vi "KonstruiereScanSteuerung.vi"(0 "VektorCluster":T2={"StartPunkt [m]"={"x"=-0.0005000005000000012, "y"=-0.0005000005000000081}, "ZeilenIncrement [m]"={"x"=0.0, "y"=0.0001}, "Zeile [m/s]"={"x"=1.0, "y"=0.0}, "Zeit/Zeile [s]"=0.001}, 1 "ParameterCluster":T4={"x Pixel"=250, "Lines"=250, "Bidirektional"=TRUE, "AD-Frequency [Hz]"=4000000.0, "Galvo Cycle [s]"=1e-05, "Smartmovedelay [s]"=0.00119, "max.accel. [m/s^2]"=270000.0}) -> (2 "ScanSteuerung":T3(array[cluster])=[{"Zeitpunkt [s]"=0.0, "Wirkung"=enum."Abs", "Kanal"=enum."SMoveTime", "Wert (/s)"=0.0008}, {"Zeitpunkt [s]"=0.0, "Wirkung"=enum."Abs", "Kanal"=enum."GalvoX", "Wert (/s)"=-0.0005000005000000012}, {"Zeitpunkt [s]"=0.0, "Wirkung"=enum."Abs", "Kanal"=enum."GalvoY", "Wert (/s)"=-0.0005000005000000081}, {"Zeitpunkt [s]"=0.0, "Wirkung"=enum."Abs", "Kanal"=enum."Galvo3", "Wert (/s)"=0.0}, {"Zeitpunkt [s]"=0.0, "Wirkung"=enum."LoopStart", "Kanal"=enum."Loop", "Wert (/s)"=10.0}, {"Zeitpunkt [s]"=0.0, "Wirkung"=enum."Inc", "Kanal"=enum."GalvoX", "Wert (/s)"=0.10000010000000015}, {"Zeitpunkt [s]"=0.0, "Wirkung"=enum."Inc", "Kanal"=enum."GalvoY", "Wert (/s)"=0.0}, {"Zeitpunkt [s]"=0.0, "Wirkung"=enum."Inc", "Kanal"=enum."Galvo3", "Wert (/s)"=51200.0}, {"Zeitpunkt [s]"=0.01, "Wirkung"=enum."Abs", "Kanal"=enum."Digital", "Wert (/s)"=1.0}, {"Zeitpunkt [s]"=0.01, "Wirkung"=enum."Inc", "Kanal"=enum."GalvoX", "Wert (/s)"=0.0}, {"Zeitpunkt [s]"=0.01, "Wirkung"=enum."Inc", "Kanal"=enum."GalvoY", "Wert (/s)"=0.6250006249999993}, {"Zeitpunkt [s]"=0.01, "Wirkung"=enum."Inc", "Kanal"=enum."Galvo3", "Wert (/s)"=0.0}, {"Zeitpunkt [s]"=0.01008, "Wirkung"=enum."Abs", "Kanal"=enum."Digital", "Wert (/s)"=0.0}, {"Zeitpunkt [s]"=0.01008, "Wirkung"=enum."Inc", "Kanal"=enum."GalvoX", "Wert (/s)"=-0.10000010000000015}, {"Zeitpunkt [s]"=0.01008, "Wirkung"=enum."Inc", "Kanal"=enum."GalvoY", "Wert (/s)"=-0.0}, {"Zeitpunkt [s]"=0.01008, "Wirkung"=enum."Inc", "Kanal"=enum."Galvo3", "Wert (/s)"=-51200.0}, {"Zeitpunkt [s]"=0.02008, "Wirkung"=enum."Abs", "Kanal"=enum."Digital", "Wert (/s)"=1.0}, {"Zeitpunkt [s]"=0.02008, "Wirkung"=enum."Inc", "Kanal"=enum."GalvoX", "Wert (/s)"=0.0}, {"Zeitpunkt [s]"=0.02008, "Wirkung"=enum."Inc", "Kanal"=enum."GalvoY", "Wert (/s)"=0.6250006249999993}, {"Zeitpunkt [s]"=0.02008, "Wirkung"=enum."Inc", "Kanal"=enum."Galvo3", "Wert (/s)"=0.0}, {"Zeitpunkt [s]"=0.02016, "Wirkung"=enum."Abs", "Kanal"=enum."Digital", "Wert (/s)"=0.0}, {"Zeitpunkt [s]"=0.02016, "Wirkung"=enum."LoopEnd", "Kanal"=enum."Loop", "Wert (/s)"=0.0}, {"Zeitpunkt [s]"=0.2016, "Wirkung"=enum."Inc", "Kanal"=enum."GalvoX", "Wert (/s)"=0.0}, {"Zeitpunkt [s]"=0.2016, "Wirkung"=enum."Inc", "Kanal"=enum."GalvoY", "Wert (/s)"=0.0}, {"Zeitpunkt [s]"=0.2016, "Wirkung"=enum."Inc", "Kanal"=enum."Galvo3", "Wert (/s)"=0.0}], 3 "Total time":dbl=0.2016, 4 "Line+Turn [s]":dbl=8e-05 format="%^#_6g")   [LabVIEW 2011]
panel:
  out "Galvo too far":cluster{"x":dbl, "y":dbl}
  out "Galvo too late time":dbl
  out "min Line+turn":dbl
  out "exactTurn [s]":dbl format="%_6g"
  out "AD/pixel":u32
  out "Pixelzeit":dbl
  out "TotalPixel":u16
  out "berechnete Umkehrzeit [s]":dbl=2.8081673263774566e-05 format="%#_4p"
  out "validTotalCycles":u32
  out "ini":T1={"Bitsize-Zwischenbild"=5.5926e-07, "CCDmin"=7850.0, "CCDscale"=-10.85, "GalvoCycle"=1.2e-05, "Ext.AD-clock"=4000000.0, "Steps per optical density"=53.33} {"CCDscale" format="%.2f"; "CCDmin" format="%.2f"; "Bitsize-Zwischenbild" format="%.2e"}
  out "Zeit [s]/zeile":dbl=0.01 min=0.0005 step=0.001 format="%^#_6g"
  out "min SMcycles":u16
  # "Used Units: Pixels or meters in the intermediate image\nchanged May 18 2011\nOld version with straight turn\nPixel,Cycles müssen an jedem Linestart synchron sein\nBerechnet die Umkehrzeit So lange, daß Pixel und SM-Cycle in der nächsten Zeile wieder synchron sind\nbi und unidirektional sind getestet"
  # "fehler: unidirektional lieferz zahlen die Smartmove runden muss: kein12ms raster! fixed??"
  # "TriggerPin0: During Turn: High (Line End)\nTriggerPin1: During Frame: High (Frame Start)"
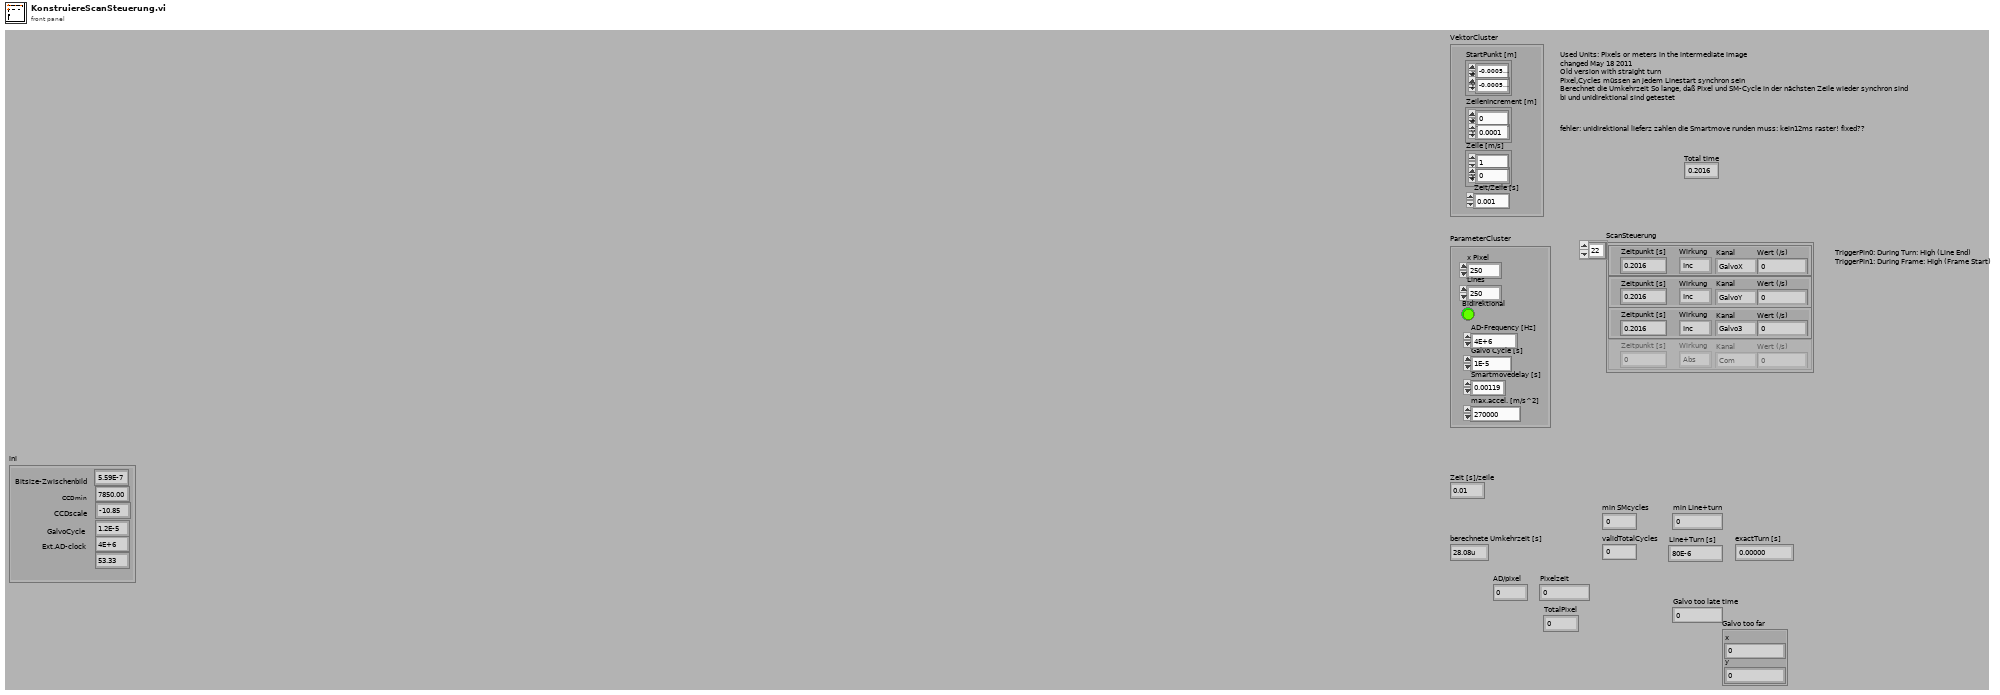
[diagram p1: front panel]
types:
  T1 = cluster{"Bitsize-Zwischenbild":dbl, "CCDmin":dbl, "CCDscale":dbl, "GalvoCycle":dbl, "Ext.AD-clock":dbl, "Steps per optical density":dbl}
  T2 = cluster{"StartPunkt [m]":cluster{"x":dbl, "y":dbl}, "ZeilenIncrement [m]":cluster{"x":dbl, "y":dbl}, "Zeile [m/s]":cluster{"x":dbl, "y":dbl}, "Zeit/Zeile [s]":dbl}
  T3 = cluster{"Zeitpunkt [s]":dbl, "Wirkung":enum16{"Abs", "Rel", "Inc", "IncInc", "LoopStart", "LoopEnd"}, "Kanal":enum16{"Com", "AnalogConfig", "AnalogValue", "GalvoX", "GalvoY", "Galvo3", "Galvo4", "Digital", "Free", "Loop", "SMoveTime", "Image1X", "Image1Y", "Image2X", "Image2Y"}, "Wert (/s)":dbl}[]
  T4 = cluster{"x Pixel":i32, "Lines":i32, "Bidirektional":bool, "AD-Frequency [Hz]":dbl, "Galvo Cycle [s]":dbl, "Smartmovedelay [s]":dbl, "max.accel. [m/s^2]":dbl}
  T5 = enum16{"Com", "AnalogConfig", "AnalogValue", "GalvoX", "GalvoY", "Galvo3", "Galvo4", "Digital", "Free", "Loop", "SMoveTime", "Image1X", "Image1Y", "Image2X", "Image2Y"}
  T6 = enum16{"Abs", "Rel", "Inc", "IncInc", "LoopStart", "LoopEnd"}
  T7 = typedef "ScanControl.ctl" = cluster{"Time [s]":dbl, "action":T8, "channel":T9, "value (/s)":dbl}[]
  T8 = typedef "ScanControl_Action.ctl" = enum16{"Abs", "Rel", "Inc", "IncInc", "LoopStart", "LoopEnd", "WaitTriggerRising"}
  T9 = typedef "ScanControl_Channel.ctl" = enum16{"Com", "AnalogConfig", "AnalogValue", "GalvoX", "GalvoY", "Galvo3", "Galvo4", "Digital", "Free", "Loop", "SMoveTime", "Image1X", "Image1Y", "Image2X", "Image2Y"}
  T10 = cluster{"Ende [s] AD+g raster":dbl, "Wirkung":enum16{"Abs", "Rel", "Inc", "IncInc", "LoopStart", "LoopEnd"}, "Kanal":enum16{"Com", "AnalogConfig", "AnalogValue", "GalvoX", "GalvoY", "Galvo3", "Galvo4", "Digital", "Free", "Loop", "SMoveTime", "Image1X", "Image1Y", "Image2X", "Image2Y"}, dbl}
  T11 = cluster{dbl, "Wirkung":enum16{"Abs", "Rel", "Inc", "IncInc", "LoopStart", "LoopEnd"}, "Kanal":enum16{"Com", "AnalogConfig", "AnalogValue", "GalvoX", "GalvoY", "Galvo3", "Galvo4", "Digital", "Free", "Loop", "SMoveTime", "Image1X", "Image1Y", "Image2X", "Image2Y"}, u8}
  T12 = cluster{dbl, "Wirkung":enum16{"Abs", "Rel", "Inc", "IncInc", "LoopStart", "LoopEnd"}, "Kanal":enum16{"Com", "AnalogConfig", "AnalogValue", "GalvoX", "GalvoY", "Galvo3", "Galvo4", "Digital", "Free", "Loop", "SMoveTime", "Image1X", "Image1Y", "Image2X", "Image2Y"}, dbl}
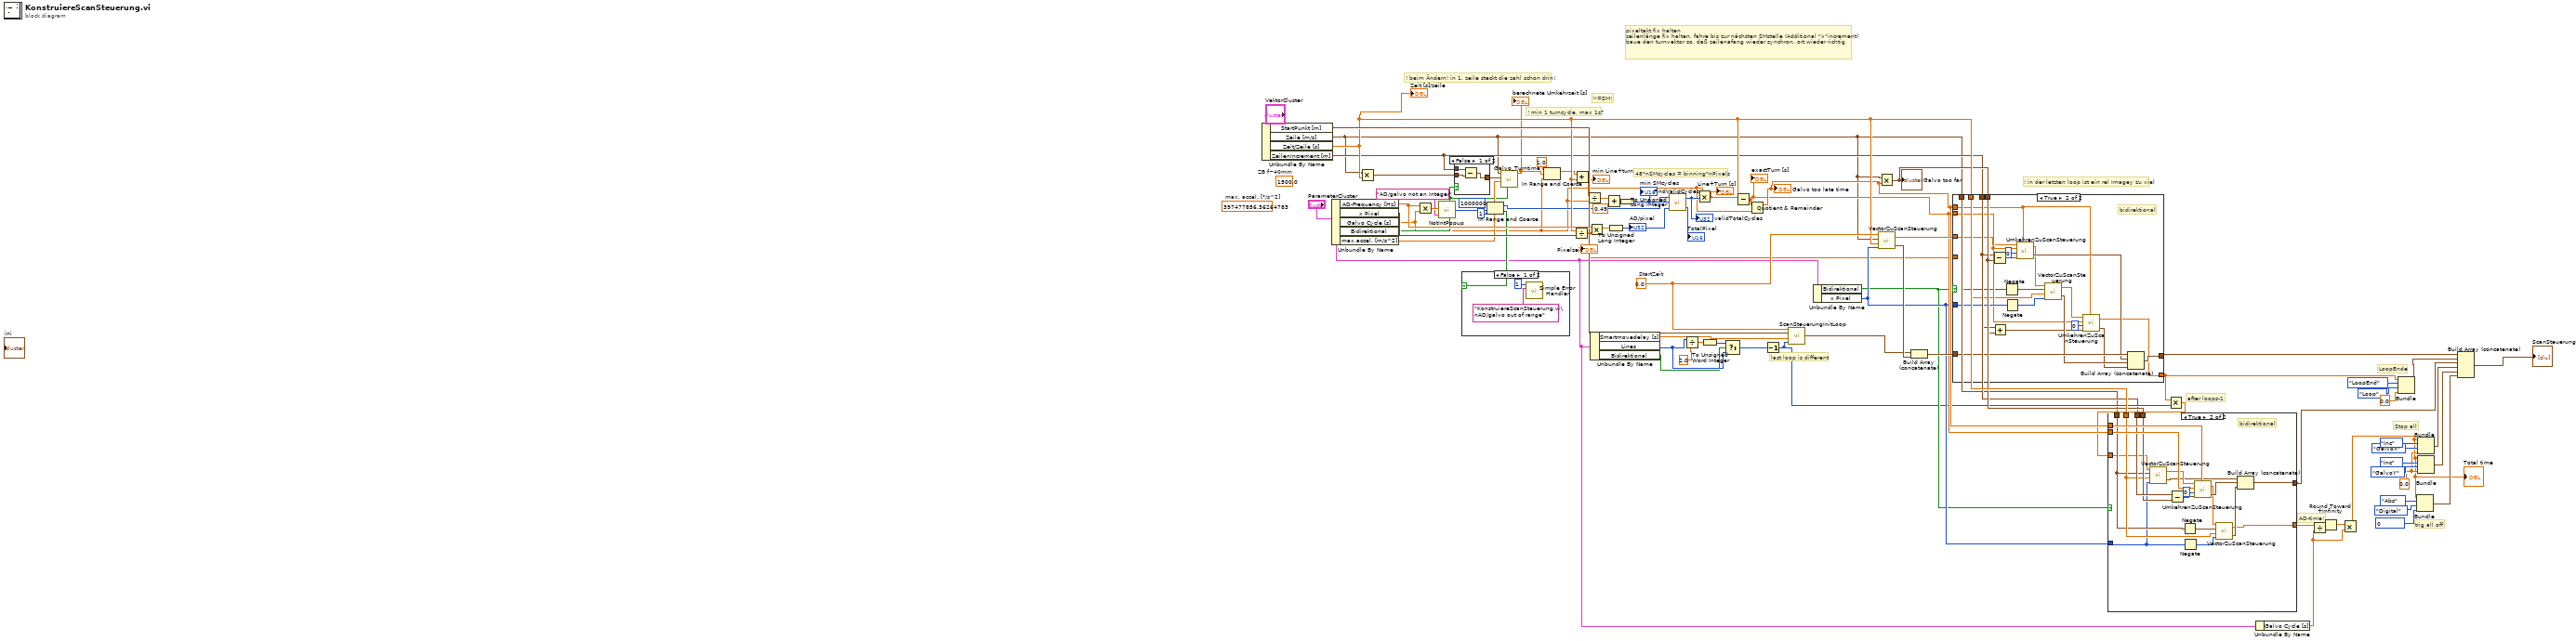
[diagram p0: block diagram]
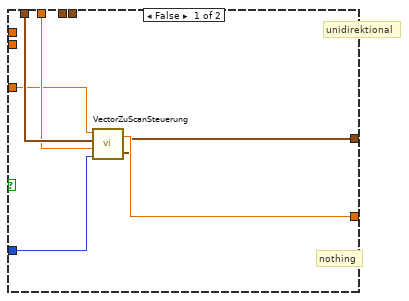
[diagram p3: hidden frame]
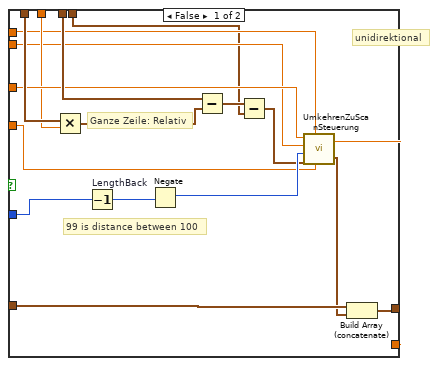
[diagram p5: hidden frame]
diagram:
  (unwired) 397477856.36264783  # max. accel. [°/s^2]
  (unwired) 1500.0  # ZB f~40mm
  w22 = 0.0
  w51 = 0.0  # StartZeit
  # "AD-time!"
  # "after loops-1"
  # "last loop is different"
  # "! in der letzten loop ist ein rel Imagey zu viel"
  # ">=SM!"
  # "! min 1 turncycle, max 1s?"
  # "pixeltakt fix halten\nzeilenlänge fix halten, fahre bis zur nächsten SMstelle (Additional \"x\"increment)\nbaue den turnvektor so, daß zeilenafang wieder synchron, ort wieder richtig"
  # "! beim Ändern! in 1. zeile steckt die zahl schon drin!"
  # "48*nSMcycles = binning*nPixels"
  # "trig all off"
  # "Stop all"
  # "LoopEnde"
  n1 = Unbundle By Name("VektorCluster") -> ("StartPunkt [m]"=w52:cluster{"x":dbl, "y":dbl}, "Zeile [m/s]"=w14:cluster{"x":dbl, "y":dbl}, "Zeit/Zeile [s]"=w45:dbl, "ZeilenIncrement [m]"=w15:cluster{"x":dbl, "y":dbl})
  "Zeit [s]/zeile" <- w45
  n2 = Unbundle By Name("ParameterCluster") -> ("AD-Frequency [Hz]"=w53:dbl, "x Pixel"=w60:i32, "Galvo Cycle [s]"=w7:dbl, "Bidirektional"=w12:bool, "max.accel. [m/s^2]"=w13:dbl)
  n3 = Multiply(x=w14, y=w45) -> (x*y=w10:cluster{"x":dbl, "y":dbl})
  n4 = Multiply(x=w53, y=w7) -> (x*y=w35:dbl)
  n5 = call "NotIntPopup.vi"("Err message"="AD/galvo not an Integer", "INT?"=w35) -> ("32bit integer"=w33:i32)  [unwired: 1 in]
  n6 = case shown="False" w12 {
    tunnel: w15 -> [w80 w81]
    tunnel: [w78 w81] -> w11
    tunnel: w10 -> [w79 _]
    frame False {
      n7 = Subtract(x=w80, y=w79) -> (x-y=w78:cluster{"x":dbl, "y":dbl})
    }
    frame True {
    }
  }
  n8 = In Range and Coerce(upper limit=1000000, x=w33, lower limit=1) -> (coerced(x)=w32:i32, In Range?=w29:bool)
  n9 = case shown="False" w29 {
    frame False {
      n10 = call <vilib>:"Simple Error Handler.vi"("error code (no error:0)"=1, "error source (\" \")"="KonstruiereScanSteuerung.vi\nAD/galvo out of range" ("Err message")) -> ()  [unwired: 2 in, 6 out]
    }
    frame True {
    }
  }
  n11 = call "Galvo_Turntime.vi"("bidirectional"=w12, "Maximal acceleration [m/s^2]"=w13, "delta x [m]"=w11, "start-speed [m/s]"=w14) -> ("duration [s]"=w6:dbl)  [unwired: 1 in, 6 out]
  "berechnete Umkehrzeit [s]" <- w6
  n12 = In Range and Coerce(upper limit=1.0, x=w6, lower limit=w7) -> (coerced(x)=w8:dbl)  [unwired: 1 out]
  n13 = Divide(x=w45, y=w60) -> (x/y=w28:dbl)
  "Pixelzeit" <- w28
  n14 = Add(x=w8, y=w45) -> (x+y=w48:dbl)
  "min Line+turn" <- w48
  n15 = Divide(x=w48, y=w7) -> (x/y=w63:dbl)
  n16 = Multiply(x=w53, y=w28) -> (x*y=w54:dbl)
  n17 = Unbundle By Name("ParameterCluster") -> ("Smartmovedelay [s]"=w50:dbl, "Lines"=w18:i32, "Bidirektional"=w17:bool)
  n18 = Add(x=w63, y=0.49) -> (x+y=w61:dbl)
  n19 = To Unsigned Long Integer(number=w54) -> (unsigned 32bit integer=w55:u32)
  "AD/pixel" <- w55
  n20 = To Unsigned Long Integer(number=w61) -> (unsigned 32bit integer=w57:u32)
  "min SMcycles" <- w57
  n21 = call "FindValidCycles.vi"("C (Fix)"=w55, "B (+x)"=w57, "A (Fix)"=w32) -> ("D"=→"TotalPixel":u32, "B Out"=w47:u32)
  "validTotalCycles" <- w47
  n22 = Divide(x=w18, y=2.0) -> (x/y=w21:dbl)
  n23 = Multiply(x=w7, y=w47) -> (x*y=w46:dbl)
  "Line+Turn [s]" <- w46
  n24 = To Unsigned Word Integer(number=w21) -> (unsigned 16bit integer=w20:u16)
  n25 = Select(t=w20, s=w17, f=w18) -> (s? t:f=w16:i32)
  n26 = Subtract(x=w46, y=w45) -> (x-y=w42:dbl)
  "exactTurn [s]" <- w42
  n27 = Quotient & Remainder(x=w42, y=w7) -> (x-y*floor(x/y)=w43:dbl)  [unwired: 1 out]
  "Galvo too late time" <- w43
  n28 = Decrement(x=w16) -> (x-1=w36:i32)
  n29 = call "ScanSteuerungInitLoop.vi"("Loops"=w36, "Smartmovedelay [s]"=w50, "StartPunkt [m]"=w52, "StartZeit"=w51) -> ("ScanSteuerung"=w49:T7)
  n30 = Unbundle By Name("ParameterCluster") -> ("Bidirektional"=w40:bool, "x Pixel"=w41:i32)
  n31 = call "VectorZuScanSteuerung.vi"("Pixel"=w41, "Zeit/zeile [s]"=w45, "Zeile [m/s]"=w14, "StartZeit"=w51) -> ("ScanSteuerung"=w59:T3, "EndZeit"=w58:dbl)
  n32 = Multiply(x=w14, y=w43) -> (x*y=w44:cluster{"x":dbl, "y":dbl})
  "Galvo too far" <- w44
  n33 = Build Array (concatenate)(w49, w59) -> (w77:T7)
  n34 = case shown="True" w40 {
    tunnel: w77 -> [w101 w123]
    tunnel: [w100 w122] -> w76
    tunnel: w14 -> [w98 w108]
    tunnel: w42 -> [w89 w116]
    tunnel: w41 -> [w86 w121]
    tunnel: w15 -> [w99 w103]
    tunnel: w45 -> [w93 w107]
    tunnel: [w97 w114] -> w68
    tunnel: w58 -> [w94 w113]
    tunnel: w43 -> [w90 w106]
    tunnel: w44 -> [w87 w102]
    tunnel: w28 -> [w85 _]
    frame False {
      # "99 is distance between 100"
      # "unidirektional"
      # "Ganze Zeile: Relativ"
      n35 = Multiply(x=w98, y=w93) -> (x*y=w91:cluster{"x":dbl, "y":dbl})
      n36 = Decrement "LengthBack"(x=w86) -> (x-1=w84:i32)
      n37 = Negate(x=w84) -> (-x=w92:i32)
      n38 = Subtract(x=w99, y=w91) -> (x-y=w96:cluster{"x":dbl, "y":dbl})
      n39 = Subtract(x=w96, y=w87) -> (x-y=w88:cluster{"x":dbl, "y":dbl})
      n40 = call "UmkehrenZuScanSteuerung.vi"("Pixeltime (only xPixel<>0)\n<Turntime?!"=w85, "Galvo too late [s]"=w90, "corrZeilenIncrement [m]"=w88, "xPixel"=w92, "Turntime [s]"=w89, "Start [s] AD raster"=w94) -> ("ScanSteuerung"=w95:T3, "Ende [s] AD+g raster"=w97:dbl)
      n41 = Build Array (concatenate)(w101, w95) -> (w100:T7)
    }
    frame True {
      # "bidirektional"
      n42 = Subtract(x=w103, y=w102) -> (x-y=w105:cluster{"x":dbl, "y":dbl})
      n43 = Add(x=w103, y=w102) -> (x+y=w104:cluster{"x":dbl, "y":dbl})
      n44 = Negate(x=w108) -> (-x=w110:cluster{"x":dbl, "y":dbl})
      n45 = Negate(x=w121) -> (-x=w109:i32)
      n46 = call "UmkehrenZuScanSteuerung.vi"("Galvo too late [s]"=w106, "corrZeilenIncrement [m]"=w105, "xPixel"=0 ("Galvo"), "Turntime [s]"=w116, "Start [s] AD raster"=w113) -> ("ScanSteuerung"=w119:T3, "Ende [s] AD+g raster"=w118:dbl)  [unwired: 1 in]
      n47 = call "VectorZuScanSteuerung.vi"("Pixel"=w109, "Zeit/zeile [s]"=w107, "Zeile [m/s]"=w110, "StartZeit"=w118) -> ("ScanSteuerung"=w120:T3, "EndZeit"=w117:dbl)
      n48 = call "UmkehrenZuScanSteuerung.vi"("Galvo too late [s]"=w106, "corrZeilenIncrement [m]"=w104, "xPixel"=0 ("Galvo"), "Turntime [s]"=w116, "Start [s] AD raster"=w117) -> ("ScanSteuerung"=w115:T3, "Ende [s] AD+g raster"=w114:dbl)  [unwired: 1 in]
      n49 = Build Array (concatenate)(w123, w119, w120, w115) -> (w122:T7)
    }
  }
  n50 = Multiply(x=w68, y=w36) -> (x*y=w39:dbl)
  n51 = case shown="True" w40 {
    tunnel: [w125 w148] -> w37
    tunnel: w14 -> [w129 w134]
    tunnel: w42 -> [_ w144]
    tunnel: w41 -> [w124 w131]
    tunnel: w15 -> [_ w138]
    tunnel: w45 -> [w128 w135]
    tunnel: [w126 w136] -> w23
    tunnel: w39 -> [w127 w133]
    tunnel: w43 -> [_ w140]
    tunnel: w44 -> [_ w137]
    frame False {
      # "nothing"
      # "unidirektional"
      n52 = call "VectorZuScanSteuerung.vi"("Pixel"=w124, "Zeit/zeile [s]"=w128, "Zeile [m/s]"=w129, "StartZeit"=w127) -> ("ScanSteuerung"=w125:T3, "EndZeit"=w126:dbl)
    }
    frame True {
      # "bidirektional"
      n53 = call "VectorZuScanSteuerung.vi"("Pixel"=w131, "Zeit/zeile [s]"=w135, "Zeile [m/s]"=w134, "StartZeit"=w133) -> ("ScanSteuerung"=w130:T3, "EndZeit"=w132:dbl)
      n54 = Subtract(x=w138, y=w137) -> (x-y=w139:cluster{"x":dbl, "y":dbl})
      n55 = Negate(x=w134) -> (-x=w142:cluster{"x":dbl, "y":dbl})
      n56 = Negate(x=w131) -> (-x=w141:i32)
      n57 = call "UmkehrenZuScanSteuerung.vi"("Galvo too late [s]"=w140, "corrZeilenIncrement [m]"=w139, "xPixel"=0 ("Galvo"), "Turntime [s]"=w144, "Start [s] AD raster"=w132) -> ("ScanSteuerung"=w146:T3, "Ende [s] AD+g raster"=w145:dbl)  [unwired: 1 in]
      n58 = call "VectorZuScanSteuerung.vi"("Pixel"=w141, "Zeit/zeile [s]"=w135, "Zeile [m/s]"=w142, "StartZeit"=w145) -> ("ScanSteuerung"=w147:T3, "EndZeit"=w136:dbl)
      n59 = Build Array (concatenate)(w130, w146, w147) -> (w148:T3)
    }
  }
  n60 = Unbundle By Name("ParameterCluster") -> ("Galvo Cycle [s]"=w1:dbl)
  n61 = Divide(x=w23, y=w1) -> (x/y=w5:dbl)
  n62 = Round Toward +Infinity(x=w5) -> (ceil(x): smallest int >= x=w2:dbl)
  n63 = Multiply(x=w2, y=w1) -> (x*y=w3:dbl)
  "Total time" <- w3
  n64 = Bundle("Ende [s] AD+g raster"=w68, "Wirkung"=T6."LoopEnd", "Kanal"=T5."Loop", 0.0) -> (w73:T10)  [unwired: 1 out]
  n65 = Bundle(w3, "Wirkung"=T6."Abs", "Kanal"=T5."Digital", u8 0) -> (w64:T11)  [unwired: 1 out]
  n66 = Bundle(w3, "Wirkung"=T6."Inc", "Kanal"=T5."GalvoX", w22) -> (w38:T12)  [unwired: 1 out]
  n67 = Bundle(w3, "Wirkung"=T6."Inc", "Kanal"=T5."GalvoY", w22) -> (w69:T12)  [unwired: 1 out]
  n68 = Build Array (concatenate)(w76, w73, w37, w38, w69, w64) -> (→"ScanSteuerung":T7)
